vi "loadModelES.vi"(0 "dl in":refnum<class "dl.lvclass">, 5 "engine model path":path, 7 "maxBatchSize":i32, 11 "error in (no error)":errorcluster) -> (4 "dl out":refnum<class "dl.lvclass">, 6 "loadESucc":i32, 15 "error out":errorcluster)   [LabVIEW 2025, in "dl.lvlib" / "dl.lvclass"]
uses:
  dl.lvclass
  dl.lvclass/dl.ctl
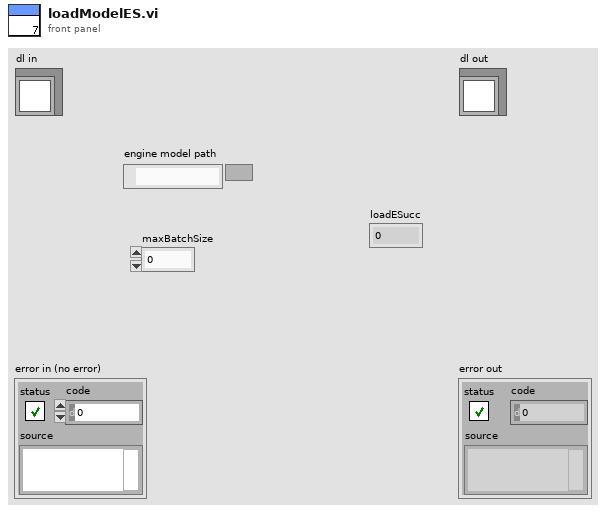
[diagram p1: front panel]
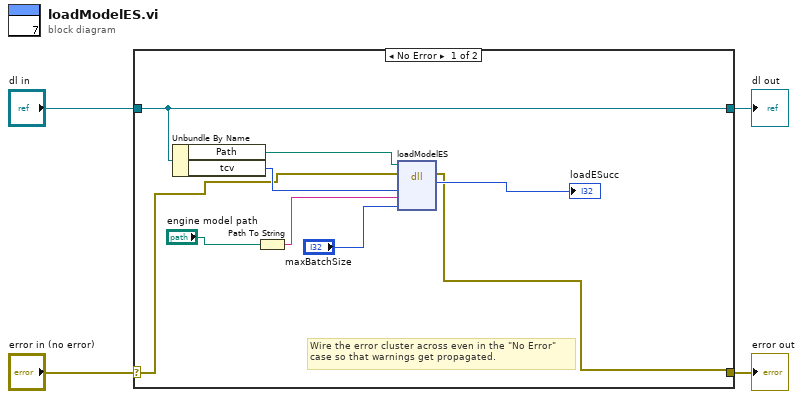
[diagram p0: block diagram]
diagram:
  n1 = case shown="No Error" "error in (no error)" {
    selector: "error in (no error)" -> [w6 w15]
    tunnel: [w5 w15] -> w3
    tunnel: [w13 w14] -> w1
    tunnel: "dl in" -> [w13 w14]
    frame No Error {
      # "Wire the error cluster across even in the \"No Error\"\ncase so that warnings get propagated."
      n2 = Unbundle By Name(w13) -> ("Path"=w12:path, "tcv"=w11:u64)
      n3 = Path To String(path="engine model path") -> (string=w9:string)
      n4 = dll-call lib="D:/Test/adslvPackageDev/Resources/TCV_Lib.dll" fn="loadModelES"(path in=w12, error in=w6, "tcv"=w11, "enginepath"=w9, "maxBatchSize"="maxBatchSize") -> (error out=w5:errorcluster, "loadESucc"=→"loadESucc":i32)  [unwired: 4 in, 1 out]
    }
    frame Error {
    }
  }
  "error out" <- w3
  "dl out" <- w1
